vi "A170316-11-Main.vi"() -> ()   [LabVIEW 2020]
uses:
  Global_Variable/Global.vi
panel:
  in  "更换产品":refnum<vi>
  out "提示信息":string
  out "错误":bool
  out "时间字符串":string
  out "日期字符串":string
  out "自动":bool
  out "判定":bool
  out "批次":bool
  out "userStatus":string caption="用户状态"
  out "userName":string caption="用户名"
  out "合格数量":dbl
  out "生产数量":dbl
  out "追溯码":string
  out "connectionMode":string caption="联机类型"
  out "产品型号":string
  in  "info":enum32{"批次", "判定"}(tab)
  in  "批次信息":string[][](table)
  in  "Result":string[][](table)
  # "总成空载力矩及啮合间隙检测台"
  # "名称"
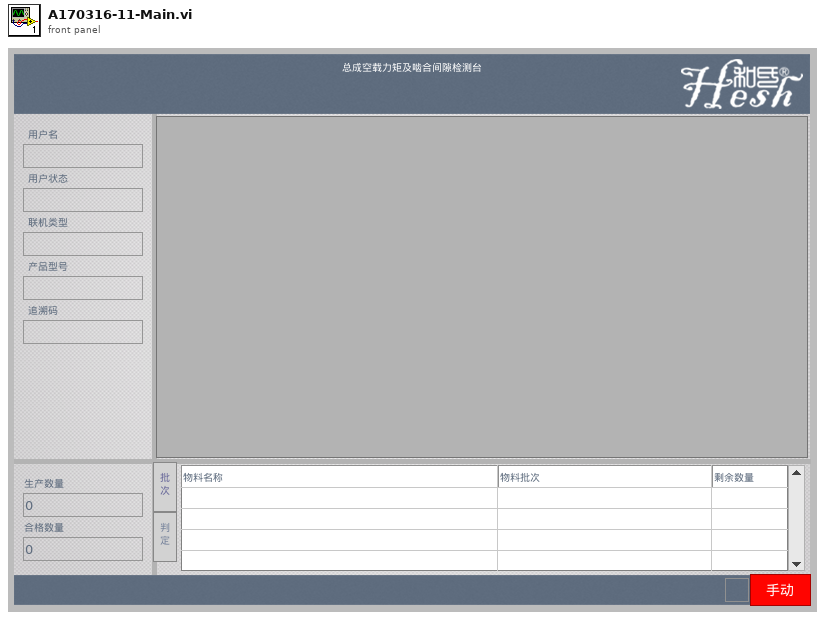
[diagram p1: front panel]
types:
  T1 = enum32{"Invalid", "Standard", "Closed", "Hidden", "Minimized", "Maximized"}
  T2 = enum32{"invalid app kind", "Development System", "Run Time System", "Student Edition", "Embedded LabVIEW", "Evaluation", "Custom"}
  T3 = cluster{"Core":cluster{"Current VI Reference":refnum<vi>, "Close Panel on Exit?":bool}, "Your Boolean data":bool, "Your string data":string}
  T4 = cluster{"Current VI Reference":refnum<vi>, "Close Panel on Exit?":bool}
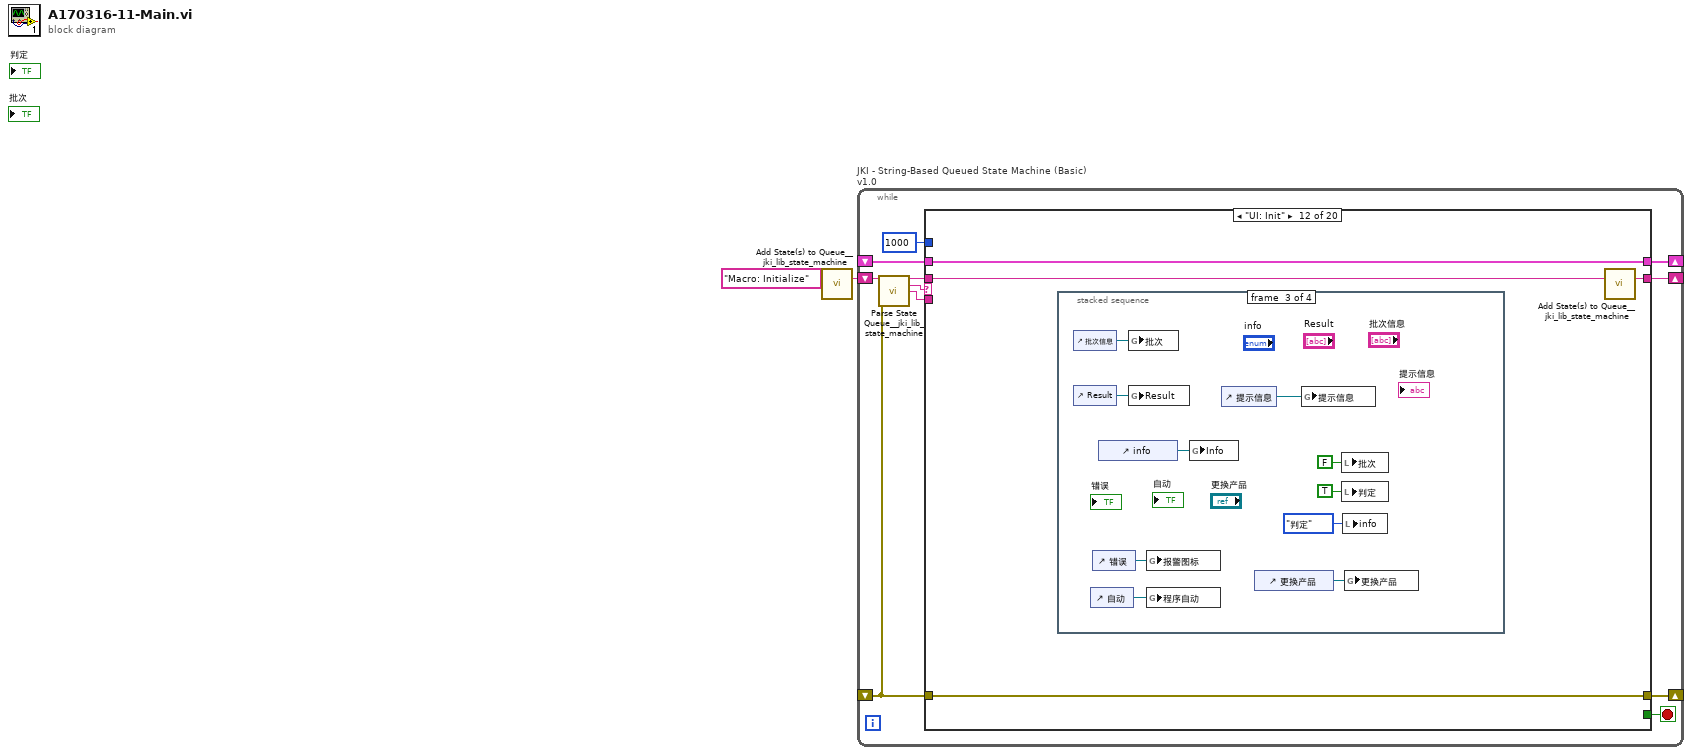
[diagram p0: block diagram]
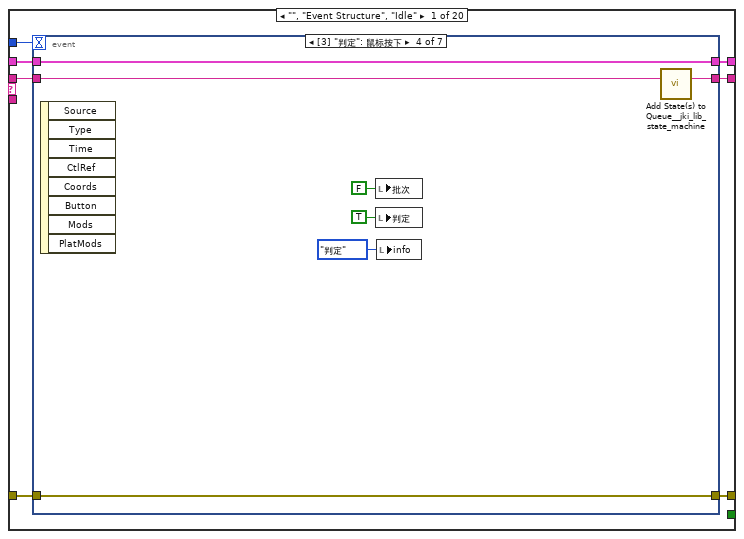
[diagram p2: hidden frame]
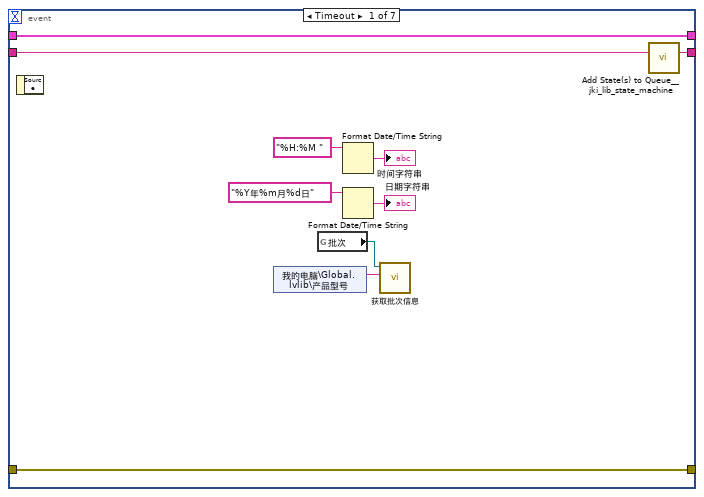
[diagram p3: hidden frame]
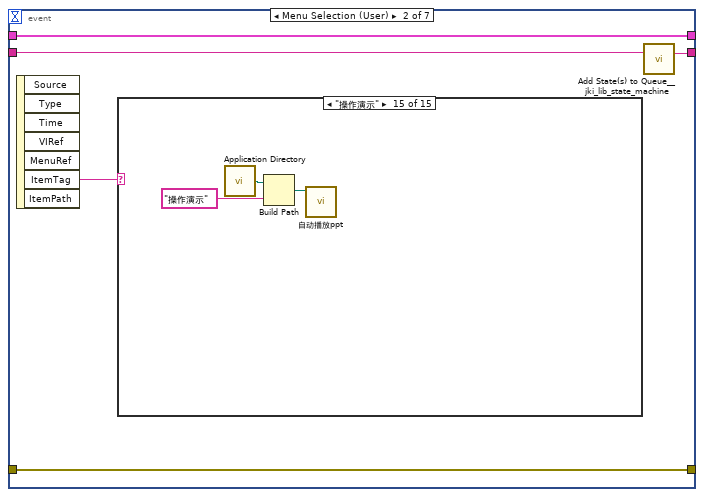
[diagram p4: hidden frame]
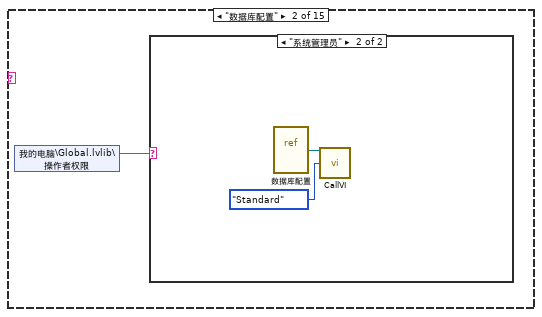
[diagram p6: hidden frame]
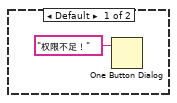
[diagram p7: hidden frame]
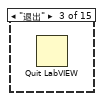
[diagram p8: hidden frame]
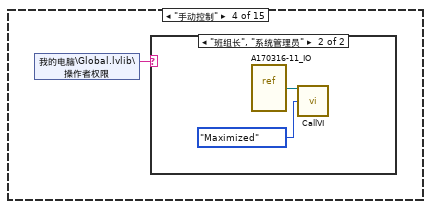
[diagram p9: hidden frame]
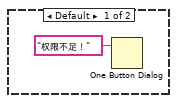
[diagram p10: hidden frame]
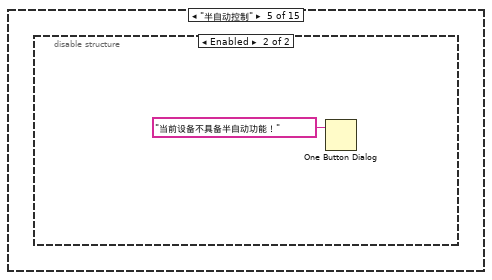
[diagram p11: hidden frame]
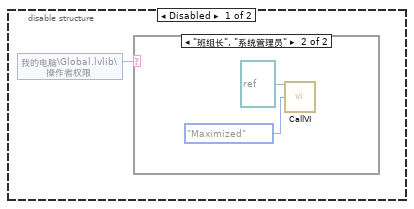
[diagram p12: hidden frame]
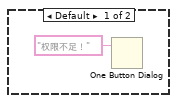
[diagram p13: hidden frame]
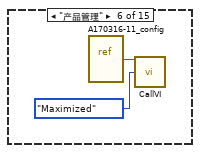
[diagram p14: hidden frame]
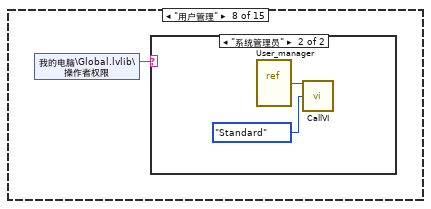
[diagram p16: hidden frame]
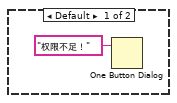
[diagram p17: hidden frame]
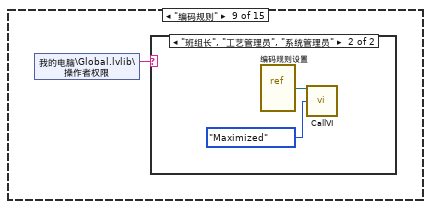
[diagram p18: hidden frame]
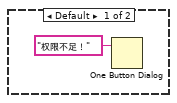
[diagram p19: hidden frame]
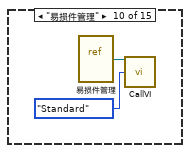
[diagram p20: hidden frame]
diagram:
  n1 = call <vilib>:"Add State(s) to Queue__jki_lib_state_machine.vi"("State(s) in (\"\")"="Macro: Initialize") -> ("States Out"=w2:string)  [unwired: 14 in]
  n2 = while "JKI - String-Based Queued State Machine (Basic) v1.0" {
    shift-right: [w6] -> _
    shift-left: _ -> [w5]
    shift-right: [w9] -> _
    shift-left: _ -> [w3]
    shift-right: [w8] -> _
    shift-left: w2 -> [w10]
    stop <- w7 stop-if-true
    n3 = call <vilib>:"Parse State Queue__jki_lib_state_machine.vi"("State Queue"=w10, "Error In (no error)"=w3) -> ("Remaining States"=w12:string, "Current State"=w13:string, "Arguments"=w11:string)  [unwired: 11 in]
    n4 = case shown="\"UI: Init\"" w13 {
      selector: w13 -> [_ _ w127 _ _ _ _ _ _ _ _ _ _ _ _ _ _ _ _ _]
      tunnel: w12 -> [w20 w126 w131 w149 w155 w160 w164 w171 w177 w181 w193 w197 w228 w239 w265 w270 w280 w284 w288 w292]
      tunnel: w11 -> [_ _ _ _ _ _ _ _ _ _ _ _ w223 w233 _ _ _ _ _ _]
      tunnel: w5 -> [w18 w123 w129 w140 w152 w158 w161 _ w172 w178 w191 w195 w226 w235 w262 w267 w277 w281 w285 w289]
      tunnel: [w17 w124 w133 w146 errorcluster {"status"=FALSE, "code"=0, "source"=""} ("error out") w157 w162 w168 w173 w179 w188 w194 w224 w236 w263 w268 w278 w282 w286 w290] -> w9
      tunnel: w3 -> [w16 w124 w132 w146 w151 w157 w162 w168 w174 w179 w184 w194 w225 w237 w263 w268 w278 w282 w286 w290]
      tunnel: [w19 w125 w130 w148 w154 w159 w163 w170 w176 w180 w192 w196 w227 w238 w264 w269 w279 w283 w287 w291] -> w8
      tunnel: [_ _ _ _ _ TRUE _ _ _ _ _ _ _ _ _ _ _ _ _ _] -> w7
      tunnel: [w15 w123 w129 w147 w152 w158 w161 w169 w172 w178 w191 w195 w226 w235 w262 w267 w277 w281 w285 w289] -> w6
      tunnel: 1000 ("Timeout") -> [w14 _ _ _ _ _ _ _ _ _ _ _ _ _ _ _ _ _ _ _]
      frame "", "Event Structure", "Idle" {
        n5 = event shown="[3] \"判定\": 鼠标按下" {
          selector: _ -> [_ _ _ _ _ _ _]
          dyn-events: _ -> [_ _ _ _ _ _ _]
          timeout: w14 -> [_ _ _ _ _ _ _]
          tunnel: w20 -> [w30 w33 w82 w93 w99 w108 w119]
          tunnel: [w29 w31 w83 w94 w100 w107 w120] -> w19
          tunnel: w18 -> [w27 w32 w84 w95 w101 w105 w122]
          tunnel: [w28 w34 w81 w92 w98 w106 w121] -> w17
          tunnel: w16 -> [w28 w34 w81 w92 w98 w106 w121]
          tunnel: [w27 w32 w84 w95 w101 w105 w122] -> w15
          event Timeout {
            n6 = event-data() -> ()  [unwired: 1 in, 1 out]
            n7 = shared-variable "我的电脑\\Global.lvlib\\产品型号"() -> (w22:string)  [unwired: 1 in, 1 out]
            n8 = global read "Global.vi" "批次"() -> (w21:refnum<vi>)
            n9 = Format Date/Time String(time format string (%c)="%H:%M ") -> (date/time string=→"时间字符串":string)  [unwired: 2 in]
            n10 = Format Date/Time String(time format string (%c)="%Y年%m月%d日") -> (date/time string=→"日期字符串":string)  [unwired: 2 in]
            n11 = call "获取批次信息.vi"("产品型号"=w22, "Tbl引用句柄"=w21) -> ()  [unwired: 8 in, 2 out]
            n12 = call <vilib>:"Add State(s) to Queue__jki_lib_state_machine.vi"("State(s) in (\"\")"=w30) -> ("States Out"=w29:string)  [unwired: 14 in]
          }
          event Menu Selection (User) {
            n13 = event-data() -> ("ItemTag"=w35:string)  [unwired: 1 in, 6 out]
            n14 = case shown="\"操作演示\"" w35 {
              frame "假", Default {
              }
              frame "数据库配置" {
                n15 = shared-variable "我的电脑\\Global.lvlib\\操作者权限"() -> (w36:string)  [unwired: 1 in, 1 out]
                n16 = case shown="\"系统管理员\"" w36 {
                  frame Default {
                    n17 = One Button Dialog(message="权限不足！" ("消息")) -> ()  [unwired: 1 in, 1 out]
                  }
                  frame "系统管理员" {
                    n18 = vi-ref "数据库配置.vi"() -> (w39:refnum<vi>)
                    n19 = call "CallVI.vi"("VI引用"=w39, "状态"=T1."Standard") -> ()  [unwired: 11 in, 3 out]
                  }
                }
              }
              frame "退出" {
                n20 = Quit LabVIEW() -> ()  [unwired: 1 in]
              }
              frame "手动控制" {
                n21 = shared-variable "我的电脑\\Global.lvlib\\操作者权限"() -> (w40:string)  [unwired: 1 in, 1 out]
                n22 = case shown="\"班组长\", \"系统管理员\"" w40 {
                  frame Default {
                    n23 = One Button Dialog(message="权限不足！" ("消息")) -> ()  [unwired: 1 in, 1 out]
                  }
                  frame "班组长", "系统管理员" {
                    n24 = vi-ref "A170316-11_IO.vi"() -> (w43:refnum<vi>)
                    n25 = call "CallVI.vi"("VI引用"=w43, "状态"=T1."Maximized") -> ()  [unwired: 11 in, 3 out]
                  }
                }
              }
              frame "半自动控制" {
                n26 = disable-structure shown="Enabled" {
                  frame Disabled {
                    n27 = shared-variable "我的电脑\\Global.lvlib\\操作者权限"() -> (w44:string)  [unwired: 1 in, 1 out]
                    n28 = case shown="\"班组长\", \"系统管理员\"" w44 {
                      frame Default {
                        n29 = One Button Dialog(message="权限不足！" ("消息")) -> ()  [unwired: 1 in, 1 out]
                      }
                      frame "班组长", "系统管理员" {
                        n30 = call "CallVI.vi"("VI引用"=refnum<vi> refnum, "状态"=T1."Maximized") -> ()  [unwired: 11 in, 3 out]
                      }
                    }
                  }
                  frame Enabled {
                    n31 = One Button Dialog(message="当前设备不具备半自动功能！" ("消息")) -> ()  [unwired: 1 in, 1 out]
                  }
                }
              }
              frame "产品管理" {
                n32 = vi-ref "A170316-11_config.vi"() -> (w50:refnum<vi>)
                n33 = call "CallVI.vi"("VI引用"=w50, "状态"=T1."Maximized") -> ()  [unwired: 11 in, 3 out]
              }
              frame "系统配置" {
              }
              frame "用户管理" {
                n34 = shared-variable "我的电脑\\Global.lvlib\\操作者权限"() -> (w51:string)  [unwired: 1 in, 1 out]
                n35 = case shown="\"系统管理员\"" w51 {
                  frame Default {
                    n36 = One Button Dialog(message="权限不足！" ("消息")) -> ()  [unwired: 1 in, 1 out]
                  }
                  frame "系统管理员" {
                    n37 = vi-ref "User_manager.vi"() -> (w54:refnum<vi>)
                    n38 = call "CallVI.vi"("VI引用"=w54, "状态"=T1."Standard") -> ()  [unwired: 11 in, 3 out]
                  }
                }
              }
              frame "编码规则" {
                n39 = shared-variable "我的电脑\\Global.lvlib\\操作者权限"() -> (w55:string)  [unwired: 1 in, 1 out]
                n40 = case shown="\"班组长\", \"工艺管理员\", \"系统管理员\"" w55 {
                  frame Default {
                    n41 = One Button Dialog(message="权限不足！" ("消息")) -> ()  [unwired: 1 in, 1 out]
                  }
                  frame "班组长", "工艺管理员", "系统管理员" {
                    n42 = vi-ref "编码规则设置.vi"() -> (w58:refnum<vi>)
                    n43 = call "CallVI.vi"("VI引用"=w58, "状态"=T1."Maximized") -> ()  [unwired: 11 in, 3 out]
                  }
                }
              }
              frame "易损件管理" {
                n44 = vi-ref "易损件管理.vi"() -> (w60:refnum<vi>)
                n45 = call "CallVI.vi"("VI引用"=w60, "状态"=T1."Standard") -> ()  [unwired: 11 in, 3 out]
              }
              frame "物料批次管理" {
                n46 = disable-structure shown="Enabled" {
                  frame Disabled {
                    n47 = vi-ref "批次管理.vi"() -> (w62:refnum<vi>)
                    n48 = call "CallVI.vi"("VI引用"=w62, "状态"=T1."Maximized") -> ()  [unwired: 11 in, 3 out]
                  }
                  frame Enabled {
                    n49 = One Button Dialog(message="当前设备无需批次管理！" ("消息")) -> ()  [unwired: 1 in, 1 out]
                  }
                }
              }
              frame "打开报表" {
                n50 = call "文件对话框"("start path"=path "D:/report", "prompt"="打开报表", "pattern (all files)"="*.doc;*.docx", "pattern label"="Word 文档") -> ("selected path"=w64:path, "error out"=w65:errorcluster)  [unwired: 8 in, 2 out]
                n51 = case shown="无错误" w65 {
                  selector: w65 -> [w71 w73]
                  tunnel: w64 -> [w72 _]
                  frame No Error {
                    w70 = 1 items=["Normal", "Maximize", "Minimize"] ("cpubbs_WindowState")
                    n52 = call "Open_Word.vi"("File Path"=w72, "cpubbs_WindowState"=w70, "错误输入（无错误）"=w71) -> ()  [unwired: 12 in, 1 out]
                  }
                  frame Error {
                    n53 = call <vilib>:"Clear Errors.vi"("error in (no error)"=w73) -> ()  [unwired: 5 in, 2 out]
                  }
                }
              }
              frame "报警信息" {
                n54 = vi-ref "报警信息.vi"() -> (w75:refnum<vi>)
                n55 = call "CallVI.vi"("VI引用"=w75, "状态"=T1."Maximized") -> ()  [unwired: 11 in, 3 out]
              }
              frame "关于" {
                n56 = vi-ref "About.vi"() -> (w77:refnum<vi>)
                n57 = call "CallVI.vi"("VI引用"=w77, "状态"=T1."Maximized") -> ()  [unwired: 11 in, 3 out]
              }
              frame "操作演示" {
                n58 = call <vilib>:"Application Directory.vi"() -> ("Application Directory"=w80:path)
                n59 = Build Path(base path=w80, name or relative path="操作演示" ("名称或相对路径")) -> (appended path=w79:path)
                n60 = call "自动播放ppt.vi"("路径"=w79) -> ()  [unwired: 10 in, 1 out]
              }
            }
            n61 = call <vilib>:"Add State(s) to Queue__jki_lib_state_machine.vi"("State(s) in (\"\")"=w33) -> ("States Out"=w31:string)  [unwired: 14 in]
          }
          event "批次": Mouse Down {
            n62 = event-data() -> ()  [unwired: 1 in, 8 out]
            n63 = disable-structure shown="禁用" {
              frame Disabled {
                n64 = local write "批次"(TRUE ("批次")) -> ()
                n65 = local write "判定"(FALSE ("判定")) -> ()
                n66 = local write "info"(enum32{"批次", "判定"}."批次" ("info")) -> ()
              }
              frame Enabled {
                n67 = One Button Dialog(message="当前设备无批次！" ("消息")) -> ()  [unwired: 1 in, 1 out]
              }
            }
            n68 = call <vilib>:"Add State(s) to Queue__jki_lib_state_machine.vi"("State(s) in (\"\")"=w82) -> ("States Out"=w83:string)  [unwired: 14 in]
          }
          event "判定": Mouse Down {
            n69 = event-data() -> ()  [unwired: 1 in, 8 out]
            n70 = local write "批次"(FALSE ("批次")) -> ()
            n71 = local write "判定"(TRUE ("判定")) -> ()
            n72 = local write "info"(enum32{"批次", "判定"}."判定" ("info")) -> ()
            n73 = call <vilib>:"Add State(s) to Queue__jki_lib_state_machine.vi"("State(s) in (\"\")"=w93) -> ("States Out"=w94:string)  [unwired: 14 in]
          }
          event "错误": Mouse Down {
            n74 = event-data() -> ()  [unwired: 1 in, 8 out]
            n75 = vi-ref "报警信息.vi"() -> (w97:refnum<vi>)
            n76 = call "CallVI.vi"("VI引用"=w97, "状态"=T1."Maximized") -> ()  [unwired: 11 in, 3 out]
            n77 = call <vilib>:"Add State(s) to Queue__jki_lib_state_machine.vi"("State(s) in (\"\")"=w99) -> ("States Out"=w100:string)  [unwired: 14 in]
          }
          event Panel Close? {
            n78 = event-data() -> ()  [unwired: 1 in, 1 out]
            n79 = global write "Global.vi" "程序关闭"(TRUE ("程序关闭")) -> ()
            n80 = event-data("Discard?"=TRUE) -> ()  [unwired: 1 in, 1 out]
            n81 = call <vilib>:"Add State(s) to Queue__jki_lib_state_machine.vi"("State(s) in Front (\"\")"="Macro: Exit", "State(s) in (\"\")"=w108) -> ("States Out"=w107:string)  [unwired: 13 in]
          }
          event "更换产品": Value Change {
            n82 = event-data() -> ("NewVal"=w118:refnum<vi>)  [unwired: 1 in, 5 out]
            n83 = property on="子面板" class="SubPnl"() -> (error out=w113:errorcluster, "InsertedVI"=w117:refnum<vi>)  [unwired: 2 in, 1 out]
            n84 = invoke class="VI" method="Abort VI"(reference=w117, error in=w113) -> (error out=w112:errorcluster)  [unwired: 1 in, 2 out]
            n85 = invoke on="子面板" class="SubPnl" method="Remove VI"(error in=w112) -> (error out=w111:errorcluster)  [unwired: 2 in, 2 out]
            n86 = Variant To Data(type=refnum<vi> refnum ("VI引用"), Variant=w118) -> (data=w109:refnum<vi>)  [unwired: 1 in, 1 out]
            n87 = invoke on="子面板" class="SubPnl" method="Insert VI"(error in=w111, "VI Ref"=w109) -> (error out=w116:errorcluster)  [unwired: 2 in, 3 out]
            n88 = invoke class="VI" method="Run VI"(reference=w109, error in=w116, "Wait until done"=FALSE ("结束前等待"), "Auto Dispose Ref"=TRUE ("自动销毁引用")) -> ()  [unwired: 1 in, 5 out]
            n89 = call <vilib>:"Add State(s) to Queue__jki_lib_state_machine.vi"("State(s) in (\"\")"=w119) -> ("States Out"=w120:string)  [unwired: 14 in]
          }
        }
      }
      frame "---------- Core ----------" {
        n90 = call <vilib>:"Add State(s) to Queue__jki_lib_state_machine.vi"("State(s) in (\"\")"=w126) -> ("States Out"=w125:string)  [unwired: 14 in]
      }
      frame Default {
        w136 = 42 items=["No error", "Argument error", "Memory is full", "Out of zone", "End of file", "File already open", "Generic file I/O error", "File not found", "File permission error", "Disk is full", "Duplicate path", "Too many files open", "System feature not enabled", "Resource file not found", "Cannot add resource", "Resource not found", "Image not found", "Image memory error", "Pen does not exist", "Config type invalid", "Config token not found", "Config parse error", "Config memory error", "Bad external code format", "Bad external code offset", "External code not present", "Null window", "Destroy window error", "Null menu", "Print aborted", "Bad print record", "Print driver error", "Windows error during printing", "Memory error during printing", "Print dialog error", "Generic print error", "Invalid device refnum", "Device not found", "Device parameter error", "Device unit error", "Cannot open device", "Device call aborted", "Generic error", "Cancelled by user", "Object ID too low", "Object ID too high", "Object not in heap", "Unknown heap", "Unknown object (invalid DefProc)", "Unknown object (DefProc not in table)", "Message out of range", "Invalid (null) method", "Unknown message", "Manager call not supported", "Bad address", "Network operation in progress", "Network operation timed out", "Connection is busy", "Network attribute not supported", "Network error", "Address in use", "System out of memory", "Connection aborted", "Connection refused", "Not connected", "Already connected", "Connection closed", "Initialization error (interapplication manager)", "Bad occurrence", "Wait on unbound occurrence handler", "Occurrence queue overflow", "Datalog type conflict", "Unused", "Unrecognized type (interapplication manager)", "Memory corrupt", "Failed to make temporary DLL", "Old CIN version", "Drag socket not found", "Failed to load drop-object", "Failed to register OLE object", "Failed to release OLE object", "Format specifier type mismatch", "Unknown format specifier", "Too few format specifiers", "Too many format specifiers", "Scan failed", "Newer CIN version", "Error converting to variant", "Runtime menu error", "Password tampered", "Variant attribute not found", "Incompatible variant data type", "Event data is not available", "Event Store is not present", "Occurrence is not found", "Event Queue is not created", "Event info is not available", "Refnum passed is NULL", "Error retrieving Class GUID", "Error retrieving CoClass GUID", "Error retrieving TypeLib GUID.", "Bad built application magic bytes.", "Specific driver is different from the specific driver associated with the Logical Name.", "There is no session opened to the class driver.", "Max Error", "MAX - Error with config objects", "MAX - Error loading configuration", "MAX - Group not supported"]
        # "Current State"
        n91 = Format Into String(format string="Software Exception: Unhandled State \"%s\"." ("message"), error in=w132, w127) -> (resulting string=w135:string, error out=w134:errorcluster)  [unwired: 1 in]
        n92 = call <vilib>:"Error Cluster From Error Code.vi"("show call chain? (False)"=TRUE, "error in (no error)"=w134, "error message (\"\")"=w135, "error code (0)"=w136) -> ("error out"=w133:errorcluster)  [unwired: 5 in]
        n93 = call <vilib>:"Add State(s) to Queue__jki_lib_state_machine.vi"("State(s) in (\"\")"=w131) -> ("States Out"=w130:string)  [unwired: 14 in]
      }
      frame "Initialize Core Data" {
        # "originally closed?"
        # "exe?"
        n94 = property class="VI"() -> ("Front Panel.Open"=w145:bool)  [unwired: 2 in, 2 out]
        n95 = property class="App"() -> ("App.Kind"=w144:T2)  [unwired: 2 in, 2 out]
        n96 = control-ref of="Current VI Reference"() -> (w138:refnum<vi>)
        n97 = Not(x=w145) -> (.not. x?=w142:bool)
        n98 = Equal?(x=w144, y=T2."Run Time System" ("Application:Kind")) -> (x = y?=w141:bool)
        n99 = Or(x=w142, y=w141) -> (x .or. y?=w139:bool)
        n100 = Bundle By Name(cluster=w140, "Core.Current VI Reference"=w138, "Core.Close Panel on Exit?"=w139) -> (w147:T3)
        n101 = call <vilib>:"Add State(s) to Queue__jki_lib_state_machine.vi"("State(s) in (\"\")"=w149) -> ("States Out"=w148:string)  [unwired: 14 in]
      }
      frame "Error Handler" {
        n102 = call <vilib>:"General Error Handler.vi"("error in (no error)"=w151) -> ()  [unwired: 10 in, 5 out]
        n103 = call <vilib>:"Add State(s) to Queue__jki_lib_state_machine.vi"("State(s) in Front (\"\")"="/* Post Error States", "State(s) in (\"\")"=w155) -> ("States Out"=w154:string)  [unwired: 13 in]
      }
      frame "Exit" {
        n104 = call <vilib>:"Add State(s) to Queue__jki_lib_state_machine.vi"("State(s) in (\"\")"=w160) -> ("States Out"=w159:string)  [unwired: 14 in]
      }
      frame "---------- Data ----------" {
        n105 = call <vilib>:"Add State(s) to Queue__jki_lib_state_machine.vi"("State(s) in (\"\")"=w164) -> ("States Out"=w163:string)  [unwired: 14 in]
      }
      frame "Data: Initialize" {
        w165 = T4 {"Current VI Reference"=refnum, "Close Panel on Exit?"=FALSE}  # Core
        w167 = TRUE  # Your Boolean data
        w166 = ""  # Your string data
        n106 = Bundle("Core"=w165, "Your Boolean data"=w167, "Your string data"=w166) -> (w169:T3)  [unwired: 1 in]
        n107 = call <vilib>:"Add State(s) to Queue__jki_lib_state_machine.vi"("State(s) in (\"\")"=w171) -> ("States Out"=w170:string)  [unwired: 14 in]
      }
      frame "Data: Cleanup" {
        n108 = Unbundle By Name(w172) -> ("Core.Current VI Reference"=w175:refnum<vi>)
        n109 = Close Reference(reference=w175, error in (no error)=w174) -> (error out=w173:errorcluster)
        n110 = call <vilib>:"Add State(s) to Queue__jki_lib_state_machine.vi"("State(s) in (\"\")"=w177) -> ("States Out"=w176:string)  [unwired: 14 in]
      }
      frame "---------- UI ----------" {
        # "Do not put any code in this frame.\n(It is a separator no-op. You can make a copy of this frame to create a new UI frame)"
        n111 = call <vilib>:"Add State(s) to Queue__jki_lib_state_machine.vi"("State(s) in (\"\")"=w181) -> ("States Out"=w180:string)  [unwired: 14 in]
      }
      frame "UI: Initialize" {
        n112 = vi-ref "选择产品.vi"() -> (w182:refnum<vi>)
        n113 = invoke on="子面板" class="SubPnl" method="Insert VI"(error in=w184, "VI Ref"=w182) -> (error out=w187:errorcluster)  [unwired: 2 in, 3 out]
        n114 = invoke class="VI" method="Run VI"(reference=w182, error in=w187, "Wait until done"=FALSE ("结束前等待"), "Auto Dispose Ref"=TRUE ("自动销毁引用")) -> (error out=w183:errorcluster)  [unwired: 1 in, 4 out]
        n115 = call "窗口自动调整.vi"("error in (no error)"=w183, "max？"=TRUE, "border spacing (2 px)"=0) -> ("error out"=w188:errorcluster)  [unwired: 3 in, 1 out]
        n116 = call <vilib>:"Add State(s) to Queue__jki_lib_state_machine.vi"("State(s) in (\"\")"=w193) -> ("States Out"=w192:string)  [unwired: 14 in]
      }
      frame "UI: Init" {
        n117 = stacked-sequence {
          frame #0 {
            w199 = FALSE ("已启用")
            n118 = Current VI's Menubar() -> (w201:refnum<k9>)
            n119 = Set Menu Item Info(7:"半自动控制" ("项标识符"), 9:w199, 11:w201) -> (0:w202:errorcluster, 3:w203:refnum<k9>)  [unwired: 4 in]
            n120 = Set Menu Item Info(7:"物料批次管理" ("项标识符"), 8:w202, 9:w199, 11:w203) -> ()  [unwired: 3 in, 2 out]
          }
          frame #1 {
            w206 = 0.0 ("合格数量")
            n121 = shared-variable "我的电脑\\Global.lvlib\\联机模式"() -> (w207:i16)  [unwired: 1 in, 1 out]
            n122 = case shown="0, 默认" w207 {
              tunnel: ["联网" ("connectionMode") "单机" ("connectionMode")] -> w208
              frame 1 {
              }
              frame 0, Default {
              }
            }
            "connectionMode" <- w208
            "生产数量" <- w206
            "合格数量" <- w206
            "追溯码" <- "" ("输出轴码")
            "产品型号" <- "" ("productsName")
          }
          frame #2 {
            n123 = control-ref of="批次信息"() -> (w220:refnum<vi>)
            n124 = control-ref of="Result"() -> (w219:refnum<vi>)
            n125 = control-ref of="自动"() -> (w213:refnum<vi>)
            n126 = control-ref of="错误"() -> (w214:refnum<vi>)
            n127 = control-ref of="info"() -> (w218:refnum<vi>)
            n128 = global write "Global.vi" "批次"(w220) -> ()
            n129 = global write "Global.vi" "Result"(w219) -> ()
            n130 = global write "Global.vi" "报警图标"(w214) -> ()
            n131 = global write "Global.vi" "程序自动"(w213) -> ()
            n132 = global write "Global.vi" "Info"(w218) -> ()
            n133 = control-ref of="提示信息"() -> (w212:refnum<vi>)
            n134 = control-ref of="更换产品"() -> (w211:refnum<vi>)
            n135 = global write "Global.vi" "提示信息"(w212) -> ()
            n136 = local write "批次"(FALSE ("批次")) -> ()
            n137 = local write "判定"(TRUE ("判定")) -> ()
            n138 = local write "info"(enum32{"批次", "判定"}."判定" ("info")) -> ()
            n139 = global write "Global.vi" "更换产品"(w211) -> ()
          }
          frame #3 {
            n140 = vi-ref "A170316-11_config.vi"() -> (w221:refnum<vi>)
            n141 = call "CallVI.vi"("VI引用"=w221, "状态"=T1."Maximized") -> ()  [unwired: 11 in, 3 out]
          }
        }
        n142 = call <vilib>:"Add State(s) to Queue__jki_lib_state_machine.vi"("State(s) in (\"\")"=w197) -> ("States Out"=w196:string)  [unwired: 14 in]
      }
      frame "UI: Cursor Set" {
        # "Argument"
        n143 = case shown="\"Idle\", 默认" w223 {
          tunnel: w225 -> [w230 w232]
          tunnel: [w229 w231] -> w224
          frame "Idle", Default {
            n144 = call <vilib>:"Unset Busy.vi"("error in (no error)"=w230) -> ("error out"=w229:errorcluster)  [unwired: 10 in]
          }
          frame "Busy" {
            n145 = call <vilib>:"Set Busy.vi"("error in (no error)"=w232) -> ("error out"=w231:errorcluster)  [unwired: 9 in, 1 out]
          }
        }
        n146 = call <vilib>:"Add State(s) to Queue__jki_lib_state_machine.vi"("State(s) in (\"\")"=w228) -> ("States Out"=w227:string)  [unwired: 14 in]
      }
      frame "UI: Front Panel State" {
        # "Argument"
        n147 = Unbundle By Name(w235) -> ("Core.Current VI Reference"=w234:refnum<vi>)
        n148 = case shown="\"Open\", 默认" w233 {
          tunnel: w237 -> [w243 w256]
          tunnel: [w245 w257] -> w236
          tunnel: w234 -> [w244 w254]
          frame "Open", Default {
            n149 = property class="VI"(reference=w244, error in=w243) -> (reference out=w241:refnum<vi>, error out=w242:errorcluster, "Front Panel.Open"=w240:bool)
            n150 = case shown="假" w240 {
              tunnel: [w248 w251] -> w245
              tunnel: w242 -> [w247 w251]
              tunnel: w241 -> [w246 _]
              frame False {
                n151 = invoke class="VI" method="FP.Open"(reference=w246, error in=w247, "Activate"=TRUE, "State"=T1."Standard") -> (error out=w248:errorcluster)  [unwired: 1 in, 4 out]
              }
              frame True {
              }
            }
          }
          frame "Close" {
            n152 = property class="VI"(reference=w254, error in=w256) -> (reference out=w253:refnum<vi>, error out=w255:errorcluster, "Front Panel.Open"=w252:bool)
            n153 = case shown="真" w252 {
              tunnel: [w258 w261] -> w257
              tunnel: w255 -> [w258 w260]
              tunnel: w253 -> [_ w259]
              frame False {
              }
              frame True {
                n154 = invoke class="VI" method="FP.Close"(reference=w259, error in=w260) -> (error out=w261:errorcluster)  [unwired: 1 in, 2 out]
              }
            }
          }
        }
        n155 = call <vilib>:"Add State(s) to Queue__jki_lib_state_machine.vi"("State(s) in (\"\")"=w239) -> ("States Out"=w238:string)  [unwired: 14 in]
      }
      frame "---------- Macro ----------" {
        n156 = call <vilib>:"Add State(s) to Queue__jki_lib_state_machine.vi"("State(s) in (\"\")"=w265) -> ("States Out"=w264:string)  [unwired: 14 in]
      }
      frame "Macro: Initialize" {
        w266 = "Data: Initialize\nInitialize Core Data\nUI: Initialize\nUI: Init\nUI: Front Panel State >> Open"  # Data: Initialize Initialize Core Data UI: Initialize UI: Init UI: Front Panel State >> Open
        n157 = call <vilib>:"Add State(s) to Queue__jki_lib_state_machine.vi"("State(s) in Front (\"\")"=w266, "State(s) in (\"\")"=w270) -> ("States Out"=w269:string)  [unwired: 13 in]
      }
      frame "Macro: Exit" {
        n158 = Unbundle By Name(w277) -> ("Core.Close Panel on Exit?"=w276:bool)
        n159 = Select(t="UI: Front Panel State >> Close", s=w276, f="") -> (s? t:f=w273:string)
        n160 = call <vilib>:"Add State(s) to Queue__jki_lib_state_machine.vi"("State(s) in (\"\")"=w273, "State(s) at Back (\"\")"="Data: Cleanup\nExit") -> ("States Out"=w271:string)  [unwired: 13 in]
        n161 = call <vilib>:"Add State(s) to Queue__jki_lib_state_machine.vi"("State(s) in Front (\"\")"=w271, "State(s) in (\"\")"=w280) -> ("States Out"=w279:string)  [unwired: 13 in]
      }
      frame "---------- New Category ----------" {
        n162 = call <vilib>:"Add State(s) to Queue__jki_lib_state_machine.vi"("State(s) in (\"\")"=w284) -> ("States Out"=w283:string)  [unwired: 14 in]
      }
      frame "New Category: 1" {
        n163 = call <vilib>:"Add State(s) to Queue__jki_lib_state_machine.vi"("State(s) in (\"\")"=w288) -> ("States Out"=w287:string)  [unwired: 14 in]
      }
      frame "New Category: 2" {
        n164 = call <vilib>:"Add State(s) to Queue__jki_lib_state_machine.vi"("State(s) in (\"\")"=w292) -> ("States Out"=w291:string)  [unwired: 14 in]
      }
    }
  }
